vi "DeBounce.vi"(10 "DB_Count":dbl, 11 "Value":bool) -> (3 "BD_Value":bool)   [LabVIEW 2016, in "ArgoBotLib.lvlib"]
uses:
  ArgoBotLib.lvlib
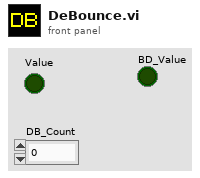
[diagram p1: front panel]
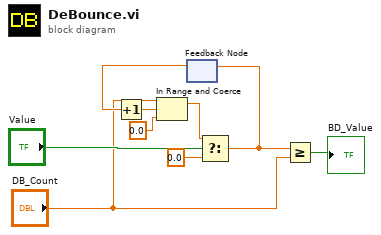
[diagram p0: block diagram]
diagram:
  n1 = feedback #1() -> (w5:dbl)  [unwired: 1 in]
  n2 = Increment(x=w5) -> (x+1=w4:dbl)
  n3 = In Range and Coerce(upper limit="DB_Count", x=w4, lower limit=0.0) -> (coerced(x)=w1:dbl)  [unwired: 1 out]
  n4 = Select(t=w1, s="Value", f=0.0) -> (s? t:f=w7:dbl)
  n5 = feedback-in #1(w7) -> ()
  n6 = Greater Or Equal?(x=w7, y="DB_Count") -> (x >= y?=→"BD_Value":bool)
